vi "json Parse Double Array - string path.vi"(8 "error in (no error)":errorcluster, 9 "default":dbl[](array[numeric]), 10 "path":string, 11 "JSON Document in":refnum<class "JSON Document.lvclass">) -> (0 "error out":errorcluster, 1 "found?":bool, 2 "value":dbl[](array[numeric]), 3 "JSON Document out":refnum<class "JSON Document.lvclass">, 4 "size":i32)   [LabVIEW 2015, in "JSON Document.lvclass"]
uses:
  JSON Document.lvclass
  JSON Document.lvclass/JSON Document.ctl
  rapidjson wrapper/rapidjson wrapper.lvlib
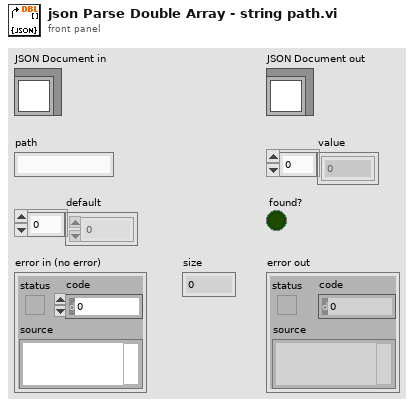
[diagram p1: front panel]
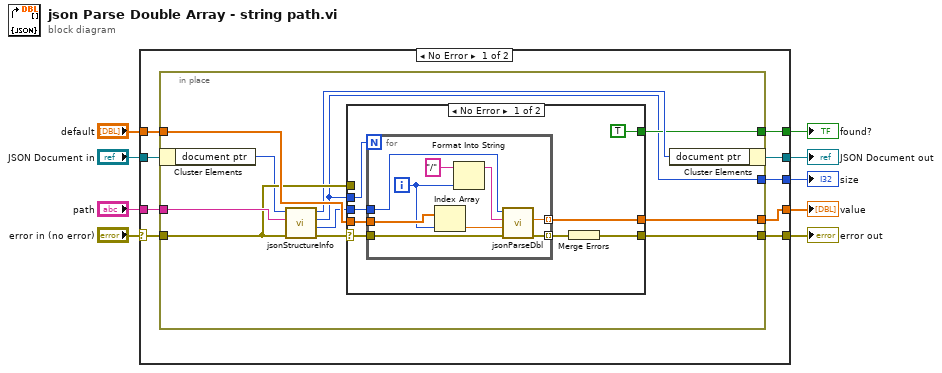
[diagram p0: block diagram]
diagram:
  n1 = case shown="No Error" "error in (no error)" {
    selector: "error in (no error)" -> [w16 w51]
    tunnel: [w15 w51] -> w8
    tunnel: [w14 w50] -> w6
    tunnel: "JSON Document in" -> [w18 w50]
    tunnel: "default" -> [w12 w49]
    tunnel: "path" -> [w17 _]
    tunnel: [w13 w49] -> w3
    tunnel: [w11 _] -> w2
    tunnel: [w10 _] -> w1
    frame No Error {
      n2 = in-place {
        in-place-border: w17 -> [w28]
        in-place-border: w16 -> [w24]
        in-place-border: [w25] -> w15
        in-place-border: [w29] -> w13
        in-place-border: w12 -> [w27]
        in-place-border: [w20] -> w11
        in-place-border: [w19] -> w10
        n3 = in-place-cluster #1(w18) -> ("document ptr"=w22:i64)
        n4 = call "jsonStructureInfo.vi"("error in (no error)"=w24, "path"=w28, "d in"=w22) -> ("error out"=w26:errorcluster, "value out"=w23:i64, "count"=w19:i32, "d out"=w21:i64)  [unwired: 5 in]
        n5 = case shown="No Error" w26 {
          selector: w26 -> [w34 _]
          tunnel: [w37 w48] -> w29
          tunnel: w19 -> [w36 _]
          tunnel: w27 -> [w35 w48]
          tunnel: [w32 w47] -> w25
          tunnel: w24 -> [_ w47]
          tunnel: w23 -> [w31 _]
          tunnel: [TRUE ("found?") _] -> w20
          frame No Error {
            n6 = for {
              N: w36 -> [_]
              tunnel: [w46] -> w33 mode=indexing
              tunnel: [w38] -> w37 mode=indexing
              tunnel: w35 -> [w42]
              tunnel: w34 -> [w43]
              tunnel: w31 -> [w39]
              i -> [w41]
              n7 = Index Array(array=w42, index=w41) -> (element=w40:dbl)
              n8 = Format Into String(initial string="/", w41) -> (resulting string=w44:string)  [unwired: 2 in, 1 out]
              n9 = call "jsonParseDbl.vi"("error in (no error)"=w43, "default"=w40, "path"=w44, "d in"=w39) -> ("error out"=w46:errorcluster, "value"=w38:dbl)  [unwired: 4 in, 2 out]
            }
            n10 = Merge Errors(w33) -> (w32:errorcluster)
          }
          frame Error {
          }
        }
        n11 = in-place-cluster #1("document ptr"=w21) -> (w14:refnum<class "JSON Document.lvclass">)
      }
    }
    frame Error {
    }
  }
  "error out" <- w8
  "JSON Document out" <- w6
  "value" <- w3
  "found?" <- w2
  "size" <- w1
